vi "Execute.vi"(8 "error in":errorcluster, 11 "SEQ in":refnum<class "SEQ.lvclass">) -> (0 "error out":errorcluster, 1 "Next Step?":bool, 2 "MSG":string, 3 "SEQ out":refnum<class "SEQ.lvclass">)   [LabVIEW 2014, in "Sequence Composition.lvlib" / "SEQ.lvclass"]
doc: "Pop the sequence stack and execute the resulting command on the sequence stack. If the command insists that we need to reinsert the current class, push it back onto the stack. If the message returned by the execution of the step is not empty, load it into the message event queue where it can be handled by the interface."
uses:
  SEQ.lvclass
  SEQ.lvclass/SEQ.ctl
  STEPS/STEP.lvclass
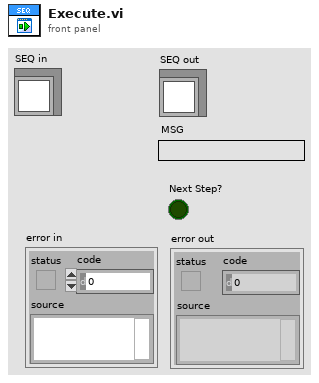
[diagram p1: front panel]
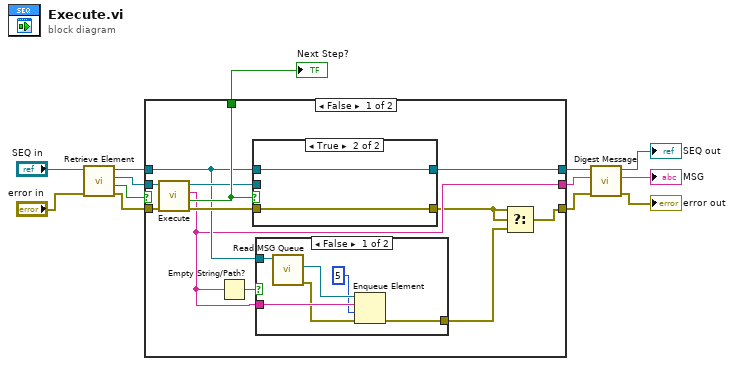
[diagram p0: block diagram]
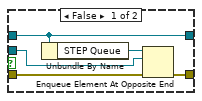
[diagram p3: hidden frame]
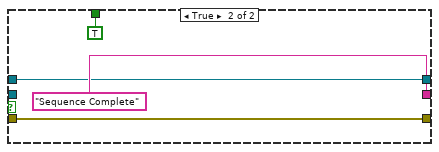
[diagram p4: hidden frame]
diagram:
  n1 = call "Retrieve Element.vi"("error in"="error in", "SEQ in"="SEQ in") -> ("error out"=w11:errorcluster, "empty?"=w7:bool, "STEP.lvclass"=w12:refnum<class "STEP.lvclass">, "SEQ out"=w13:refnum<class "SEQ.lvclass">)  [unwired: 6 in]
  n2 = case shown="False" w7 {
    tunnel: w13 -> [w19 w40]
    tunnel: [w25 w40] -> w5
    tunnel: [w15 w39] -> w2
    tunnel: w12 -> [w23 _]
    tunnel: w11 -> [w22 w39]
    tunnel: [w21 TRUE ("Next Step?")] -> w10
    tunnel: [w17 "Sequence Complete" ("t")] -> w6
    frame False {
      n3 = call-dynamic "Execute.vi"("error in"=w22, "STEP in"=w23) -> ("error out"=w24:errorcluster, "Next Step?"=w21:bool, "MSG"=w17:string, "STEP out"=w20:refnum<class "STEP.lvclass">)  [unwired: 6 in]
      n4 = Empty String/Path?(string/path=w17) -> (empty?=w18:bool)
      n5 = case shown="True" w21 {
        tunnel: w19 -> [w33 w38]
        tunnel: [w33 w38] -> w25
        tunnel: w24 -> [w32 w37]
        tunnel: [w35 w37] -> w16
        tunnel: w20 -> [w34 _]
        frame False {
          n6 = Unbundle By Name(w33) -> ("STEP Queue"=w36:refnum<queue>)
          n7 = Enqueue Element At Opposite End(queue=w36, element=w34, error in (no error)=w32) -> (error out=w35:errorcluster)  [unwired: 1 in, 2 out]
        }
        frame True {
        }
      }
      n8 = case shown="False" w18 {
        tunnel: w19 -> [w30 _]
        tunnel: w17 -> [w31 _]
        tunnel: [w28 _] -> w14
        frame False {
          n9 = call "Read MSG Queue.vi"("SEQ in"=w30) -> ("error out"=w27:errorcluster, "MSG Queue"=w29:refnum<queue>)  [unwired: 8 in, 1 out]
          n10 = Enqueue Element(queue=w29, element=w31, timeout in ms (-1)=5, error in (no error)=w27) -> (error out=w28:errorcluster)  [unwired: 2 out]
        }
        frame True {
        }
      }
      n11 = Select(t=w16, s=w16, f=w14) -> (s? t:f=w15:errorcluster)
    }
    frame True {
    }
  }
  "Next Step?" <- w10
  n12 = call "Digest Message.vi"("error in (no error)"=w2, "MSG"=w6, "SEQ in"=w5) -> ("error out"=→"error out":errorcluster, "MSG Out"=→"MSG":string, "SEQ out"=→"SEQ out":refnum<class "SEQ.lvclass">)  [unwired: 6 in]
